vi "LED.vi"() -> ()   [LabVIEW 2020]
uses:
  <vilib>/numeric/Random Number (Range) DBL.vi
panel:
  out "error out":errorcluster
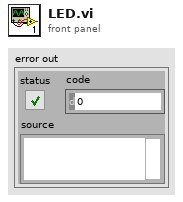
[diagram p1: front panel]
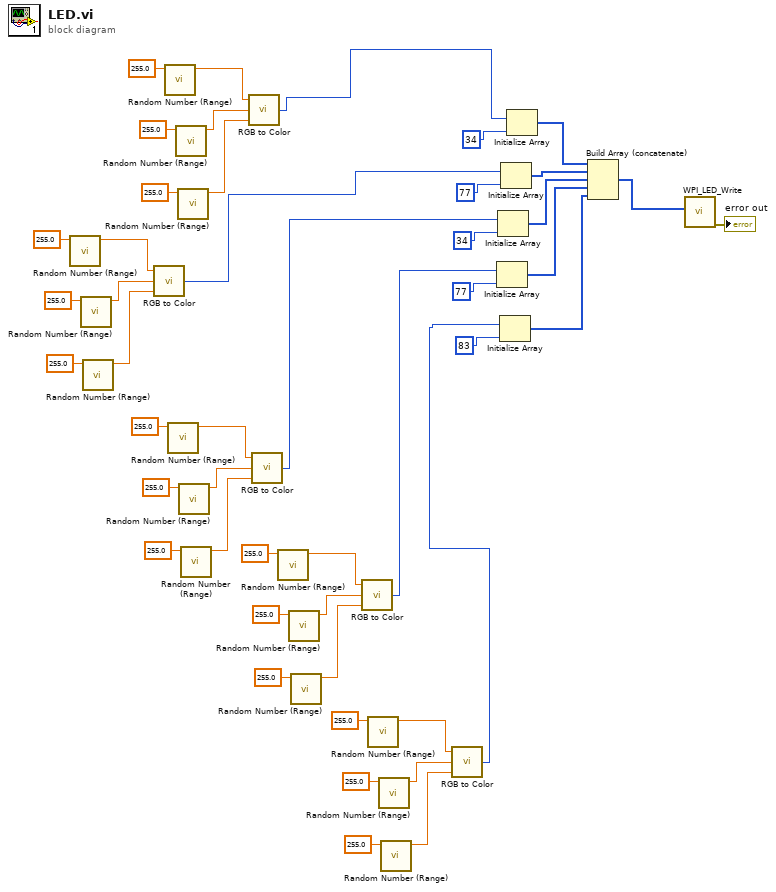
[diagram p0: block diagram]
diagram:
  n1 = call-poly <vilib>:"Random Number (Range).vi"("upper bound (100)"=255.0) -> ("number"=w24:dbl)  [unwired: 10 in]
  n2 = call-poly <vilib>:"Random Number (Range).vi"("upper bound (100)"=255.0) -> ("number"=w25:dbl)  [unwired: 10 in]
  n3 = call-poly <vilib>:"Random Number (Range).vi"("upper bound (100)"=255.0) -> ("number"=w26:dbl)  [unwired: 10 in]
  n4 = call <vilib>:"RGB to Color.vi"("B"=w26, "G"=w25, "R"=w24) -> ("Color"=w2:u32)
  n5 = call-poly <vilib>:"Random Number (Range).vi"("upper bound (100)"=255.0) -> ("number"=w31:dbl)  [unwired: 10 in]
  n6 = call-poly <vilib>:"Random Number (Range).vi"("upper bound (100)"=255.0) -> ("number"=w18:dbl)  [unwired: 10 in]
  n7 = call-poly <vilib>:"Random Number (Range).vi"("upper bound (100)"=255.0) -> ("number"=w32:dbl)  [unwired: 10 in]
  n8 = call-poly <vilib>:"Random Number (Range).vi"("upper bound (100)"=255.0) -> ("number"=w33:dbl)  [unwired: 10 in]
  n9 = call-poly <vilib>:"Random Number (Range).vi"("upper bound (100)"=255.0) -> ("number"=w19:dbl)  [unwired: 10 in]
  n10 = call-poly <vilib>:"Random Number (Range).vi"("upper bound (100)"=255.0) -> ("number"=w20:dbl)  [unwired: 10 in]
  n11 = call <vilib>:"RGB to Color.vi"("B"=w33, "G"=w32, "R"=w31) -> ("Color"=w30:u32)
  n12 = call <vilib>:"RGB to Color.vi"("B"=w20, "G"=w19, "R"=w18) -> ("Color"=w3:u32)
  n13 = call-poly <vilib>:"Random Number (Range).vi"("upper bound (100)"=255.0) -> ("number"=w12:dbl)  [unwired: 10 in]
  n14 = call-poly <vilib>:"Random Number (Range).vi"("upper bound (100)"=255.0) -> ("number"=w13:dbl)  [unwired: 10 in]
  n15 = call-poly <vilib>:"Random Number (Range).vi"("upper bound (100)"=255.0) -> ("number"=w14:dbl)  [unwired: 10 in]
  n16 = call <vilib>:"RGB to Color.vi"("B"=w14, "G"=w13, "R"=w12) -> ("Color"=w4:u32)
  n17 = call-poly <vilib>:"Random Number (Range).vi"("upper bound (100)"=255.0) -> ("number"=w6:dbl)  [unwired: 10 in]
  n18 = call-poly <vilib>:"Random Number (Range).vi"("upper bound (100)"=255.0) -> ("number"=w7:dbl)  [unwired: 10 in]
  n19 = call-poly <vilib>:"Random Number (Range).vi"("upper bound (100)"=255.0) -> ("number"=w8:dbl)  [unwired: 10 in]
  n20 = call <vilib>:"RGB to Color.vi"("B"=w8, "G"=w7, "R"=w6) -> ("Color"=w5:u32)
  n21 = Initialize Array(w4, 77 ("dimension size")) -> (w38:u32[])
  n22 = Initialize Array(w3, 34 ("dimension size")) -> (w41:u32[])
  n23 = Initialize Array(w5, 83 ("dimension size")) -> (w37:u32[])
  n24 = Initialize Array(w2, 77 ("dimension size")) -> (w1:u32[])
  n25 = Initialize Array(w30, 34 ("dimension size")) -> (w44:u32[])
  n26 = Build Array (concatenate)(w44, w1, w41, w38, w37) -> (w45:u32[])
  n27 = call <vilib>:"WPI_LED_Write.vi"("Color Array"=w45) -> ("error out"=→"error out":errorcluster)  [unwired: 10 in]
